vi "GT Set Wait Pulse Ex.vi"(7 "waitPulseDuty":dbl, 8 "error in (no error)":errorcluster caption="错误输入（无错误）", 9 "waitPulseFrq":dbl, 10 "mode":u16, 11 "cardNum":i16) -> (0 "error out":errorcluster caption="错误输出", 3 "function return":i16)   [LabVIEW 2014, in "gts.lvlib"]
doc: "GT_API GT_SetWaitPulseEx(short cardNum,unsigned short mode,double waitPulseFrq,double waitPulseDuty);"
uses:
  gts.lvlib
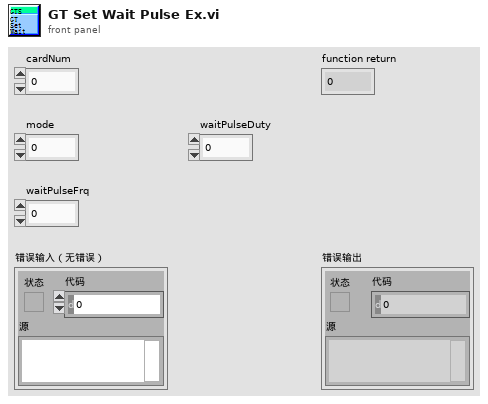
[diagram p1: front panel]
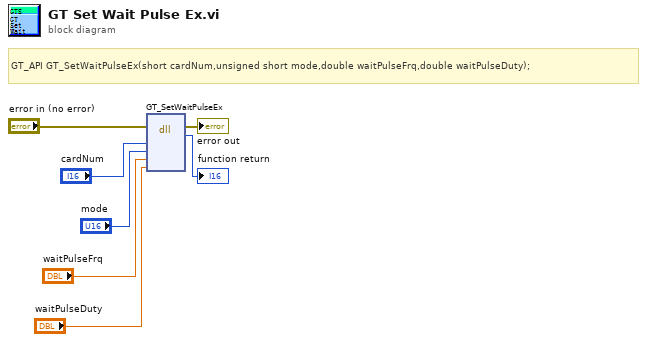
[diagram p0: block diagram]
diagram:
  # "GT_API GT_SetWaitPulseEx(short cardNum,unsigned short mode,double waitPulseFrq,double waitPulseDuty);"
  n1 = dll-call lib="PTH2habs D固高科技资料GTS控制卡GTS卡18年上半年资料dllVC32bit\nmulti_cardgts.*" fn="GT_SetWaitPulseEx"(error in="error in (no error)", "cardNum"="cardNum", "mode"="mode", "waitPulseFrq"="waitPulseFrq", "waitPulseDuty"="waitPulseDuty") -> (error out=→"error out":errorcluster, →"function return":i16)  [unwired: 6 in, 1 out]
